vi "Message generator.vi"(7 "cash":i32, 8 "error in":errorcluster, 9 "correct pin":bool=TRUE, 10 "Customer":T3, 11 "order":T1) -> (0 "error out":errorcluster, 1 "Right Menu":T2, 2 "Left Menu":T2, 3 "message":string)   [LabVIEW 2015]
uses:
  Controls/User data.ctl
  Controls/#status message.ctl
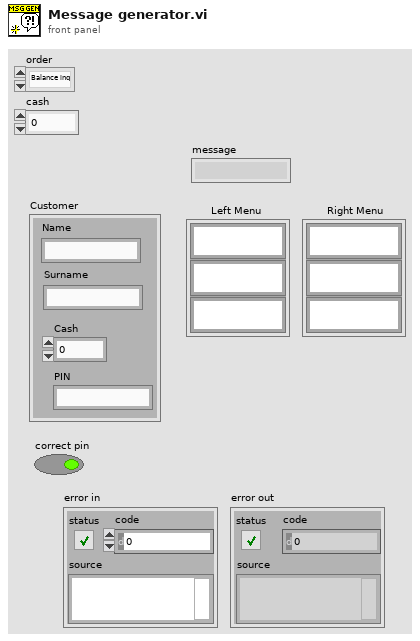
[diagram p1: front panel]
types:
  T1 = typedef "#status message.ctl" = enum16{"Balance inq", "Withdraw welcome", "Withdraw Failed", "Deposit welcome", "End of Time", "Show messsage", "Check PIN", "Initialize", "Exit", "Return&Terminate", "Balance Inquiry", "None", "First Cash", "Withdraw", "Deposit"}
  T2 = cluster{"RFS String":string, "RFS String 2":string, "RFS String 3":string}
  T3 = typedef "User data.ctl" = cluster{"Name":string, "Surname":string, "Cash":i32, "PIN":string}
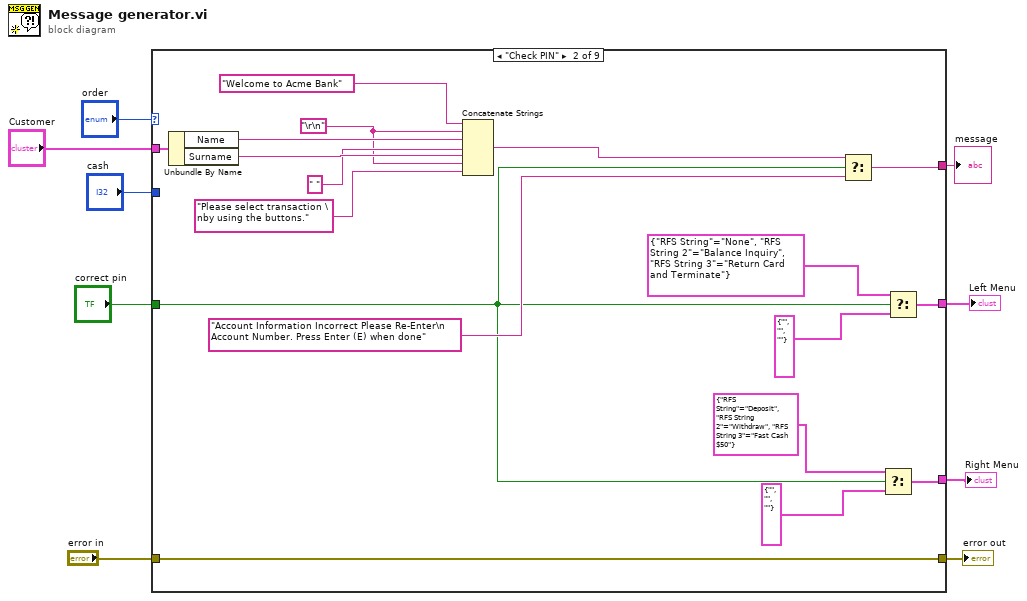
[diagram p0: block diagram]
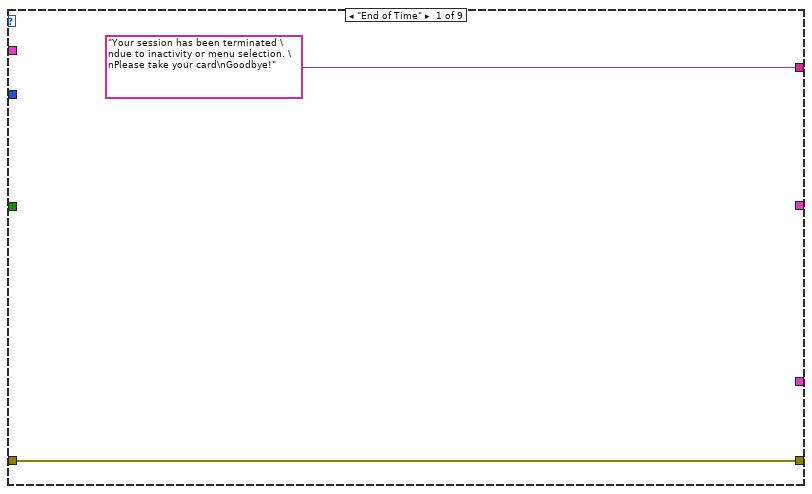
[diagram p2: hidden frame]
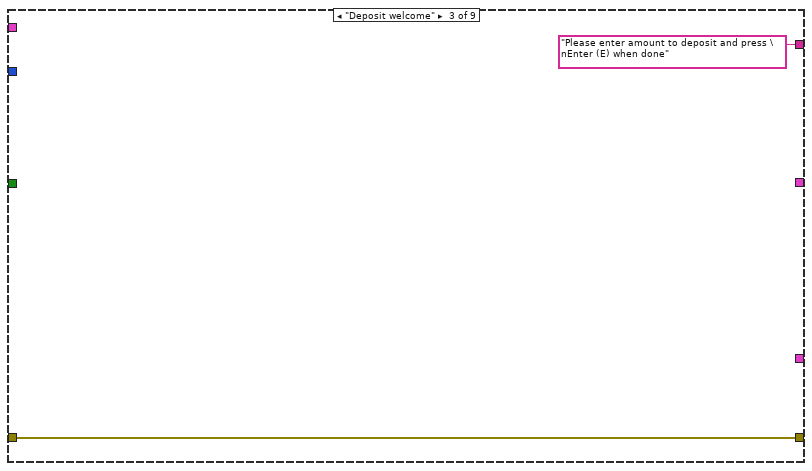
[diagram p3: hidden frame]
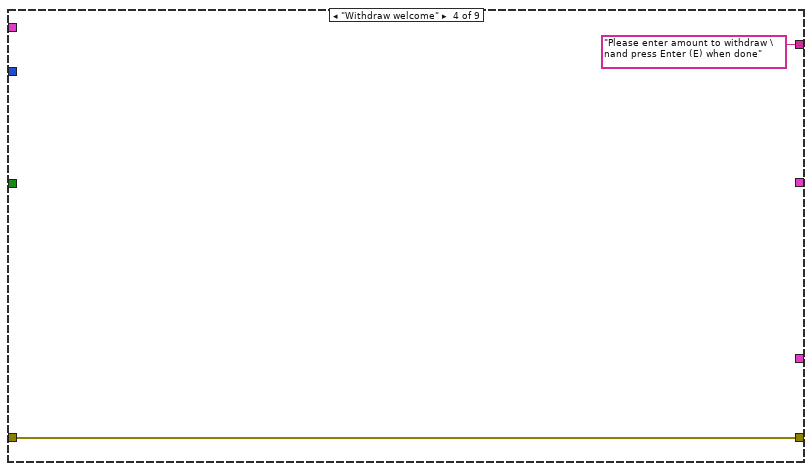
[diagram p4: hidden frame]
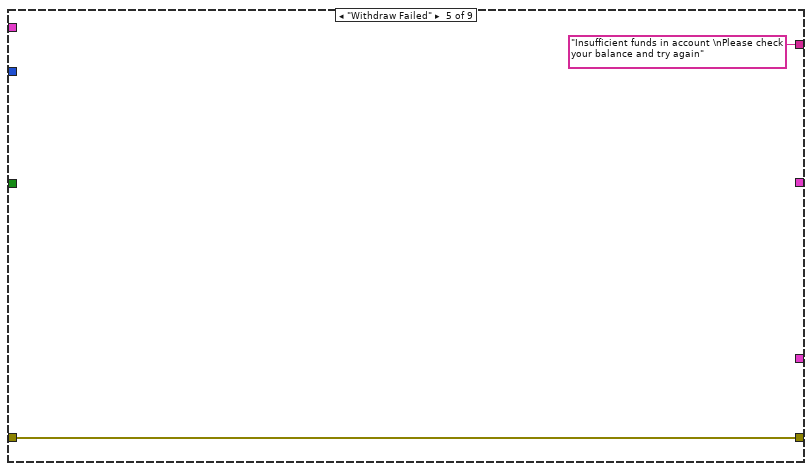
[diagram p5: hidden frame]
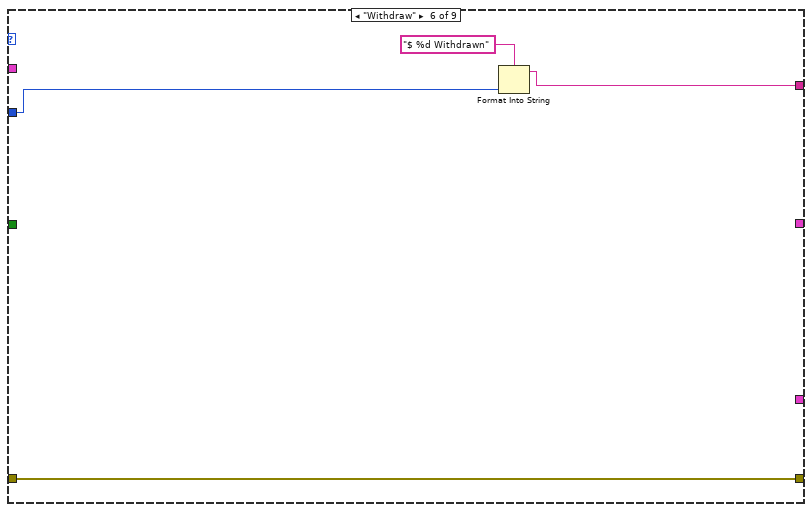
[diagram p6: hidden frame]
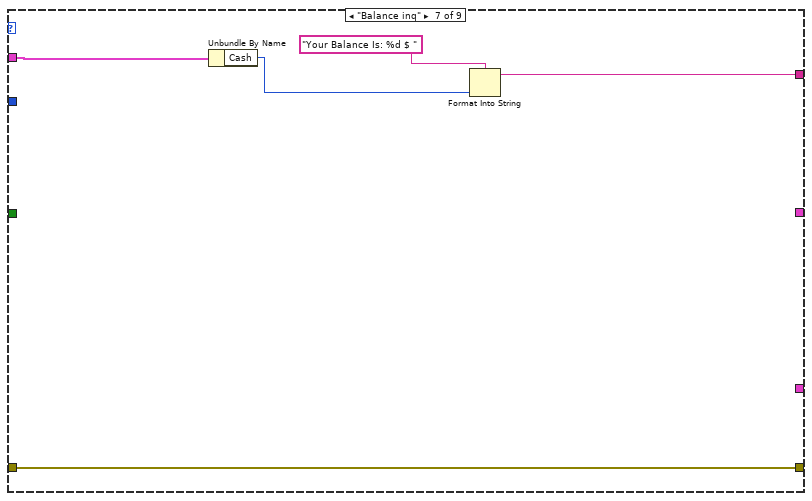
[diagram p7: hidden frame]
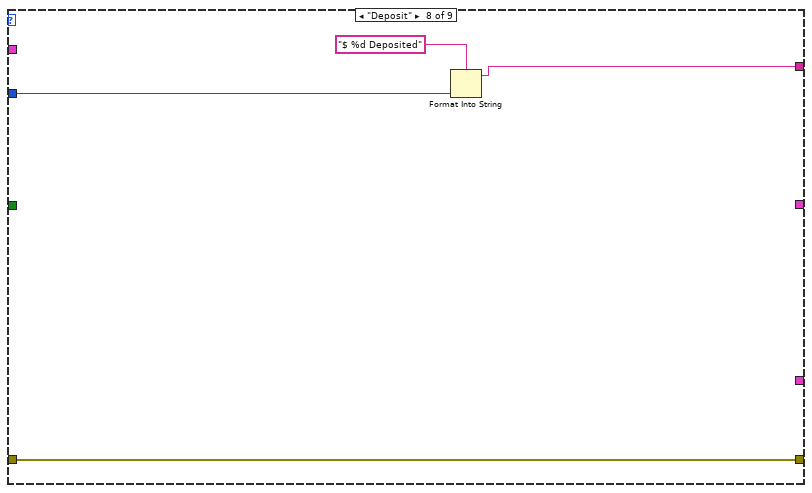
[diagram p8: hidden frame]
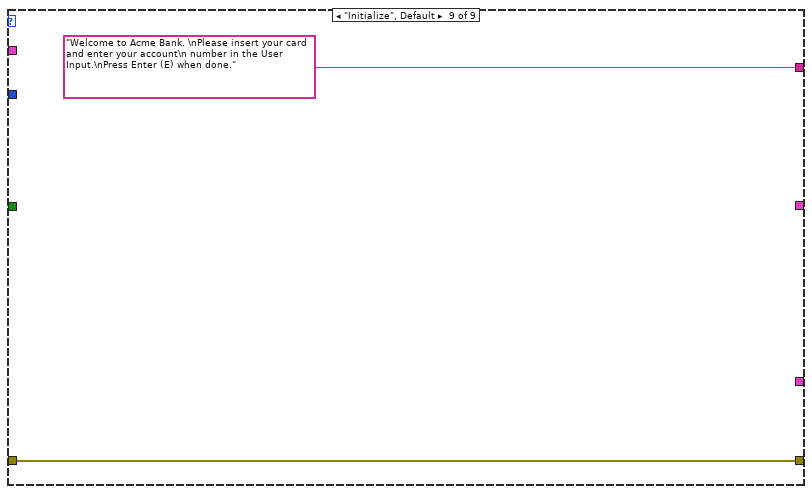
[diagram p9: hidden frame]
diagram:
  n1 = case shown="\"Check PIN\"" "order" {
    tunnel: ["Your session has been terminated \ndue to inactivity or menu selection. \nPlease take your card\nGoodbye!" ("Message") w22 "Please enter amount to deposit and press \nEnter (E) when done" ("Message") "Please enter amount to withdraw \nand press Enter (E) when done" ("Message") "Insufficient funds in account \nPlease check your balance and try again" ("Message") w39 w40 w48 "Welcome to Acme Bank. \nPlease insert your card and enter your account\n number in the User Input.\nPress Enter (E) when done."] -> w7
    tunnel: "correct pin" -> [_ w21 _ _ _ _ _ _ _]
    tunnel: "Customer" -> [_ w25 _ _ _ _ w44 _ _]
    tunnel: [_ w15 _ _ _ _ _ _ _] -> w6
    tunnel: [_ w16 _ _ _ _ _ _ _] -> w5
    tunnel: [w10 w14 w30 w33 w35 w38 w43 w47 w49] -> w4
    tunnel: "error in" -> [w10 w14 w30 w33 w35 w38 w43 w47 w49]
    tunnel: "cash" -> [_ _ _ _ _ w37 _ w46 _]
    frame "End of Time" {
    }
    frame "Check PIN" {
      w13 = "\r\n"
      n2 = Unbundle By Name(w25) -> ("Name"=w24:string, "Surname"=w28:string)
      n3 = Concatenate Strings("Welcome to Acme Bank" ("string"), w13, w24, " " ("string"), w28, w13, "Please select transaction \nby using the buttons." ("string")) -> (w23:string)
      n4 = Select(t=w23, s=w21, f="Account Information Incorrect Please Re-Enter\n Account Number. Press Enter (E) when done") -> (s? t:f=w22:string)
      n5 = Select(t=T2 {"RFS String"="Deposit", "RFS String 2"="Withdraw", "RFS String 3"="Fast Cash $50"} ("Right Menu"), s=w21, f=T2 {"RFS String"="", "RFS String 2"="", "RFS String 3"=""} ("Right Menu")) -> (s? t:f=w16:T2)
      n6 = Select(t=T2 {"RFS String"="None", "RFS String 2"="Balance Inquiry", "RFS String 3"="Return Card and Terminate"} ("Left Menu"), s=w21, f=T2 {"RFS String"="", "RFS String 2"="", "RFS String 3"=""} ("Left Menu")) -> (s? t:f=w15:T2)
    }
    frame "Deposit welcome" {
    }
    frame "Withdraw welcome" {
    }
    frame "Withdraw Failed" {
    }
    frame "Withdraw" {
      n7 = Format Into String(format string="$ %d Withdrawn" ("initial string"), w37) -> (resulting string=w39:string)  [unwired: 2 in, 1 out]
    }
    frame "Balance inq" {
      n8 = Unbundle By Name(w44) -> ("Cash"=w42:i32)
      n9 = Format Into String(format string="Your Balance Is: %d $ " ("string"), w42) -> (resulting string=w40:string)  [unwired: 2 in, 1 out]
    }
    frame "Deposit" {
      n10 = Format Into String(format string="$ %d Deposited" ("Message"), w46) -> (resulting string=w48:string)  [unwired: 2 in, 1 out]
    }
    frame "Initialize", Default {
    }
  }
  "message" <- w7
  "error out" <- w4
  "Left Menu" <- w6
  "Right Menu" <- w5
